vi "Rotate Angle in Radians (Scalar).vi"(7 "output range (-pi to pi)":T1=enum."-pi to pi", 9 "ccw rotation (rad)":dbl, 11 "angle in (rad)":dbl) -> (3 "angle out (rad)":dbl)   [LabVIEW 2017, in "NI_Robotics Utilities.lvlib"]
doc: "This VI is deprecated. Use <vi.lib>\\Analysis\\coordinate.llb\\Angle Rotation.vi instead."
uses:
  <vilib>/robotics/Utilities/NI_Robotics Utilities.lvlib
  <vilib>/robotics/Utilities/Angle Range_Radians.ctl
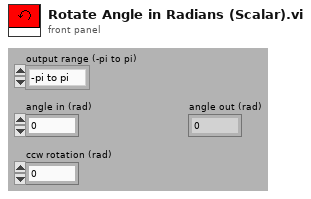
[diagram p1: front panel]
types:
  T1 = typedef "NI_Robotics Utilities.lvlib/Angle Range_Radians.ctl" = enum16{"none", "-pi to pi", "0 to 2*pi"}
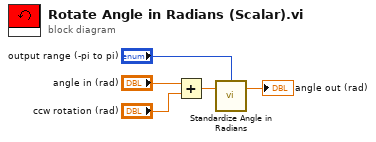
[diagram p0: block diagram]
diagram:
  n1 = Add(x="angle in (rad)", y="ccw rotation (rad)") -> (x+y=w3:dbl)
  n2 = call <vilib>:"Standardize Angle in Radians.vi"("angle in (rad)"=w3, "range (-pi to pi)"="output range (-pi to pi)") -> ("angle out (rad)"=→"angle out (rad)":dbl)  [unwired: 3 in]
